vi "subStage_MoveAbs.vi"(7 "Stage Info":T2={" Current Position"=[-1.0, -12.0, 0.0], "Number of Axis"=3, "ILSID"=1}, 8 "error in (no error)":errorcluster, 11 "Stage-Ctrl":T1={"Console"={"L"=FALSE, "R"=FALSE, "FWD"=FALSE, "BACK"=FALSE}, "Step Width [mm]"=1.0, "Destination [mm]"=[6.0, 7.0], "Move "=FALSE} {"Destination [mm]" format="%_6g"; "Step Width [mm]" min=0.0 format="%_6f"}) -> (0 "error out":errorcluster)   [LabVIEW 2015]
panel:
  # "X"
  # "Y"
  # "X"
  # "Y"
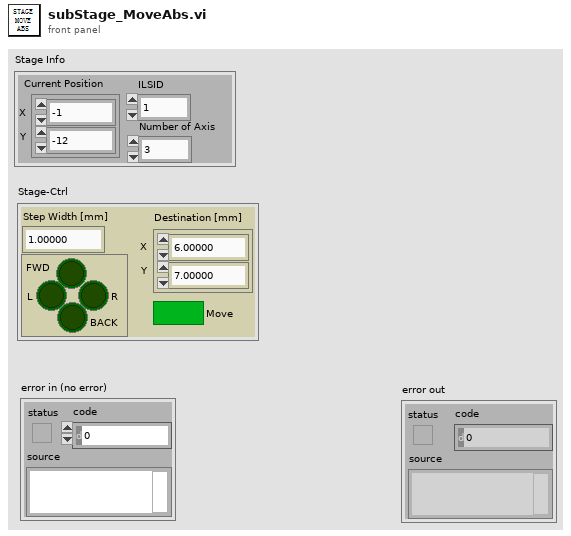
[diagram p1: front panel]
types:
  T1 = cluster{"Console":cluster{"L":bool, "R":bool, "FWD":bool, "BACK":bool}, "Step Width [mm]":dbl, "Destination [mm]":dbl[], "Move ":bool}
  T2 = cluster{" Current Position":dbl[], "Number of Axis":i32, "ILSID":i32}
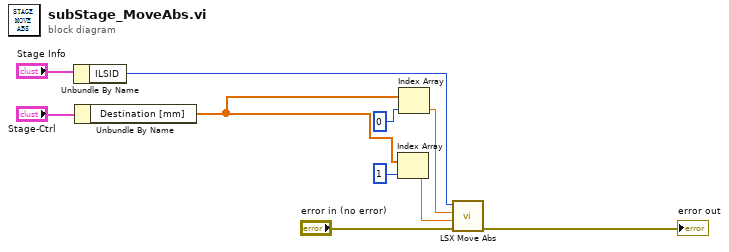
[diagram p0: block diagram]
diagram:
  n1 = Unbundle By Name("Stage Info") -> ("ILSID"=w6:i32)
  n2 = Unbundle By Name("Stage-Ctrl") -> ("Destination [mm]"=w2:dbl[])
  n3 = Index Array(array=w2, index=1) -> (element=w3:dbl)
  n4 = Index Array(array=w2, index=0) -> (element=w4:dbl)
  n5 = call <userlib>:"LSX Move Abs.vi"("error in (no error)"="error in (no error)", "dY"=w3, "dX"=w4, "lLSID"=w6) -> ("error out"=→"error out":errorcluster)  [unwired: 6 in, 1 out]
